vi "ACC_LabVIEW_RevisionQuery.vi"() -> (0 "Instrument Firmware Revision":string, 1 "Instrument Driver Revision":string)   [LabVIEW 2014, in "ACC_LabVIEW.lvlib"]
uses:
  ACC_LabVIEW.lvlib
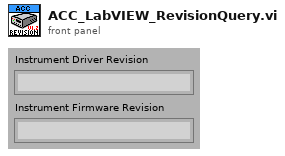
[diagram p1: front panel]
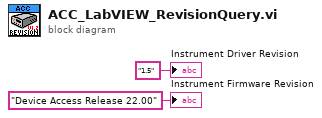
[diagram p0: block diagram]
diagram:
  "Instrument Driver Revision" <- "1.5" ("Instrument Driver Revision")
  "Instrument Firmware Revision" <- "Device Access Release 22.00" ("Instrument Firmware Revision")
